vi "waveformFromArray.vi"(10 "sample_freq":i32, 11 "Array":dbl[](array[numeric])) -> (3 "waveform":waveform(dbl))   [LabVIEW 2017]
uses:
  <vilib>/Waveform/WDTOps.llb/WDT Scale Delta t DBL.vi
panel:
  out "waveform out":waveform(dbl)
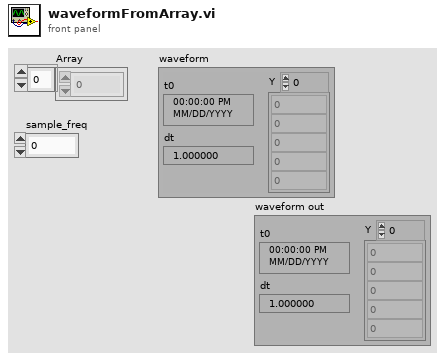
[diagram p1: front panel]
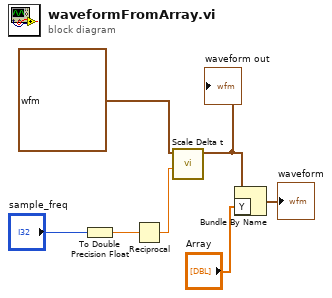
[diagram p0: block diagram]
diagram:
  n1 = To Double Precision Float(number="sample_freq") -> (double precision float=w4:dbl)
  n2 = Reciprocal(x=w4) -> (1/x=w3:dbl)
  n3 = call-poly <vilib>:"Scale Delta t.vi"("scale factor"=w3, "waveform in"=waveform(dbl) {"t0"=timestamp(0 s since 1904-01-01), "dt"=1.0, "Y"=[]} ("waveform")) -> ("waveform out"=w1:waveform(dbl))  [unwired: 8 in, 1 out]
  "waveform out" <- w1
  n4 = Bundle By Name(cluster=w1, "Y"="Array") -> (→"waveform":waveform(dbl))
